vi "SLSC Convert ENUM Value to ENUM String.vi"(11 "enums":T1[](array[typedef])) -> (3 "string enums":T3(array[cluster]))   [LabVIEW 2017, in "SLSC Tree Control.lvlib"]
doc: "Converts the ENUM datatype into ENUM strings used in the SLSC Output Tree control."
uses:
  SLSC Tree Control.lvlib
  Ctrl/EnumValue.ctl
  Ctrl/Enum.ctl
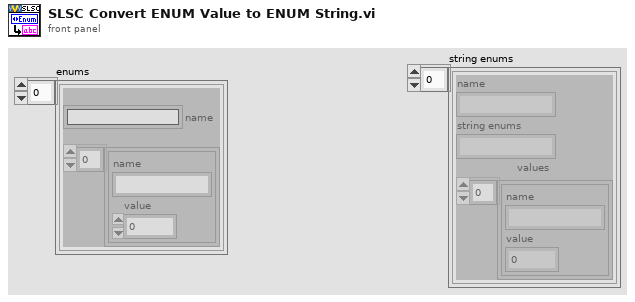
[diagram p1: front panel]
types:
  T1 = typedef "Enum.ctl" = cluster{"name":string, "values":T2[]}
  T2 = typedef "EnumValue.ctl" = cluster{"name":string, "value":i32}
  T3 = cluster{"name":string, "string enums":string, "values":T2[]}[]
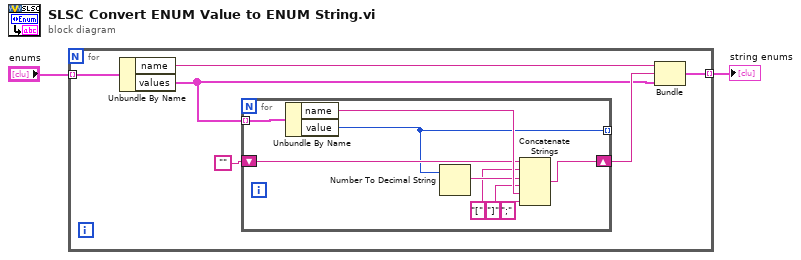
[diagram p0: block diagram]
diagram:
  n1 = for {
    tunnel: "enums" -> [w8] mode=indexing
    tunnel: [w4] -> w2 mode=indexing
    n2 = Unbundle By Name(w8) -> ("name"=w5:string, "values"=w3:T2[])
    n3 = for {
      tunnel: w3 -> [w10] mode=indexing
      shift-right: [w16] -> w6
      shift-left: "" -> [w15]
      tunnel: [w9] -> _ mode=indexing
      n4 = Unbundle By Name(w10) -> ("name"=w17:string, "value"=w9:i32)
      n5 = Number To Decimal String(number=w9) -> (decimal integer string=w14:string)  [unwired: 1 in]
      n6 = Concatenate Strings(w15, "[" ("string"), w14, "]" ("string"), w17, ";" ("string")) -> (w16:string)
    }
    n7 = Bundle("name"=w5, w6, "values"=w3) -> (w4:cluster{"name":string, string, "values":T2[]})  [unwired: 1 in]
  }
  "string enums" <- w2
